vi "CuLab_Windowing_SGL.vi"(7 "window":u16(ring) items=["None "=0, "Hanning"=1, "Hamming"=2, "Blackman-Harris"=3, "Exact Blackman"=4, "Blackman"=5, "Flat Top"=6, "4 Term B-Harris "=7, "7 Term B-Harris"=8, "Low Sidelobe"=9, "Blackman Nuttall"=11], 8 "error in (no error)":errorcluster, 11 "T1D_SGL in":refnum<class "T1D_SGL.lvclass">) -> (0 "error out":errorcluster, 3 "T1D_SGL out":refnum<class "T1D_SGL.lvclass">)   [LabVIEW 2020]
uses:
  <vilib>/Ngene/CuLab - GPU Accelerated Toolkit/Toolkit/Low_Level/Tensor_Classes/T_Children/T1D/T1D_Children/T1D_SGL/T1D_SGL.lvclass
  C:/Program Files/National Instruments/LabVIEW 2020/vi.lib/Ngene/CuLab - GPU Accelerated Toolkit/Toolkit/Low_Level/Tensor_Classes/T_Children/T1D/T1D.lvclass
  C:/Program Files/National Instruments/LabVIEW 2020/vi.lib/Ngene/CuLab - GPU Accelerated Toolkit/Toolkit/Low_Level/Tensor_Classes/Tensor.lvclass
  93686d1c-d6de-4b16-a0fc-7f36ed8a1a68.vi
  0b8842e4-a500-4db8-ba12-85dbe126322b.vi
  <vilib>/Ngene/CuLab - GPU Accelerated Toolkit/Toolkit/API/Array/Array Size/CU_Array_Size_T1D.vi
  <vilib>/Ngene/CuLab - GPU Accelerated Toolkit/Toolkit/Low_Level/Tensor_Classes/T_Children/T1D/T1D_Children/T1D_SGL/Create_Push.vi
  <vilib>/Ngene/CuLab - GPU Accelerated Toolkit/Toolkit/API/Numeric/Multiply/T1D/CU_Multiply_T1D_SGL.vi
  <vilib>/Ngene/CuLab - GPU Accelerated Toolkit/Toolkit/CuLab.lvlib
  <vilib>/Analysis/NI_AALPro.lvlib
  C:/Program Files/National Instruments/LabVIEW 2020/vi.lib/Ngene/CuLab - GPU Accelerated Toolkit/Toolkit/Low_Level/Tensor_Classes/T_Children/T1D/T1D_Children/T1D_SGL/T1D_SGL.lvclass
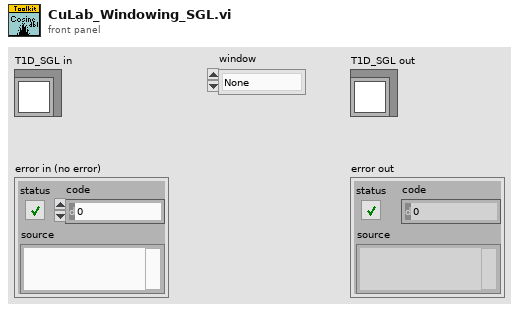
[diagram p1: front panel]
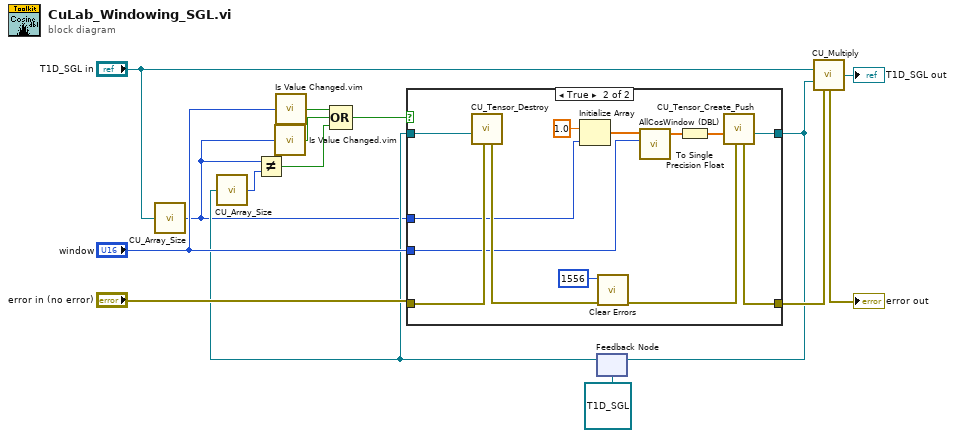
[diagram p0: block diagram]
diagram:
  n1 = call-poly <vilib>:"CU_Array_Size.vi"("Tensor"="T1D_SGL in") -> ("size"=w2:i32)  [unwired: 14 in]
  n2 = call "Is Value Changed.vim"("value"=w2) -> ("changed or first call?"=w8:bool)
  n3 = call "Is Value Changed.vim"("value"="window") -> ("changed or first call?"=w10:bool)
  n4 = feedback #1(refnum<class "T1D_SGL.lvclass"> refnum ("Dest out")) -> (w4:refnum<class "T1D_SGL.lvclass">)
  n5 = call-poly <vilib>:"CU_Array_Size.vi"("Tensor"=w4) -> ("size"=w3:i32)  [unwired: 14 in]
  n6 = Not Equal?(x=w2, y=w3) -> (x != y?=w1:bool)
  n7 = Compound Arithmetic op=OR(w10, w8, w1) -> (w9:bool)
  n8 = case shown="True" w9 {
    tunnel: w4 -> [w17 w29]
    tunnel: "error in (no error)" -> [w16 w28]
    tunnel: "window" -> [_ w27]
    tunnel: [w16 w20] -> w11
    tunnel: [w17 w25] -> w5
    tunnel: w2 -> [_ w23]
    frame False {
    }
    frame True {
      n9 = call <vilib>:"CU_Tensor_Destroy.vi"("error in (no error)"=w28, "Tensor in"=w29) -> ("error out"=w30:errorcluster)  [unwired: 9 in]
      n10 = Initialize Array(1.0 ("element"), w23) -> (w21:dbl[])
      n11 = call <vilib>:"Clear Errors.vi"("error in (no error)"=w30, "specific error code to clear (0: all)"=1556) -> ("error out"=w19:errorcluster)  [unwired: 4 in, 1 out]
      n12 = call <vilib>:"AllCosWindow (DBL).vi"("window"=w27, "X"=w21) -> ("Windowed X"=w26:dbl[])  [unwired: 3 in, 1 out]
      n13 = To Single Precision Float(number=w26) -> (single precision float=w24:sgl[])
      n14 = call-poly <vilib>:"CU_Tensor_Create_Push.vi"("error in (no error)"=w19, "CPU_Data_1D_SGL"=w24) -> ("T1D_SGL out"=w25:refnum<class "T1D_SGL.lvclass">, "error out"=w20:errorcluster)  [unwired: 8 in]
    }
  }
  n15 = feedback-in #1(w5) -> ()
  n16 = call-poly <vilib>:"CU_Multiply.vi"("x"="T1D_SGL in", "y"=w5, "error in (no error)"=w11) -> ("Dest out"=→"T1D_SGL out":refnum<class "T1D_SGL.lvclass">, "error out"=→"error out":errorcluster)  [unwired: 11 in]
